vi "Write Conversion Time.vi"(8 "error in":errorcluster, 10 "conversion time":T1, 11 "thermocouple mode in":refnum<class "Thermocouple Mode.lvclass">) -> (0 "error out":errorcluster, 3 "thermocouple mode out":refnum<class "Thermocouple Mode.lvclass">)   [LabVIEW 2017, in "Scan Engine Scripting.lvlib" / "Thermocouple Mode.lvclass"]
uses:
  Thermocouple Mode.lvclass
  Conversion Time.ctl
  Thermocouple Mode.lvclass/Thermocouple Mode.ctl
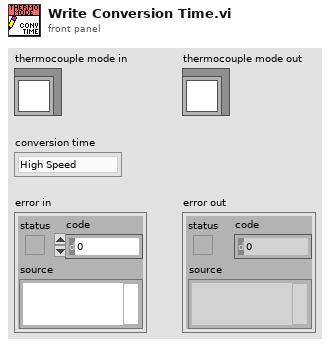
[diagram p1: front panel]
types:
  T1 = typedef "Scan Engine Scripting.lvlib/Thermocouple Mode.lvclass/Conversion Time.ctl" = enum16{"High Speed", "High Resolution"}
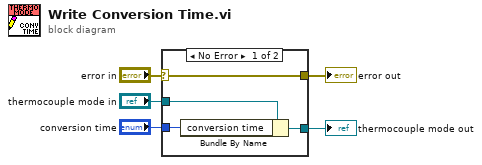
[diagram p0: block diagram]
diagram:
  n1 = case shown="No Error" "error in" {
    selector: "error in" -> [w9 w10]
    tunnel: [w9 w10] -> w4
    tunnel: [w7 w11] -> w2
    tunnel: "thermocouple mode in" -> [w8 w11]
    tunnel: "conversion time" -> [w6 _]
    frame No Error {
      n2 = Bundle By Name(cluster=w8, "conversion time"=w6) -> (w7:refnum<class "Thermocouple Mode.lvclass">)
    }
    frame Error {
    }
  }
  "error out" <- w4
  "thermocouple mode out" <- w2
